vi "PFI-28000-Base_Get VISA.vi"(8 "error in (no error)":errorcluster, 11 "PFI-28000-Base in":refnum<class "PFI-28000-Base.lvclass">) -> (0 "error out":errorcluster, 2 "VISA":refnum<visa-resource-name>, 3 "PFI-28000-Base out":refnum<class "PFI-28000-Base.lvclass">)   [LabVIEW 2017, in "PFI-28000-Base.lvclass"]
uses:
  PFI-28000-Base.lvclass
  PFI-28000-Base.lvclass/PFI-28000-Base.ctl
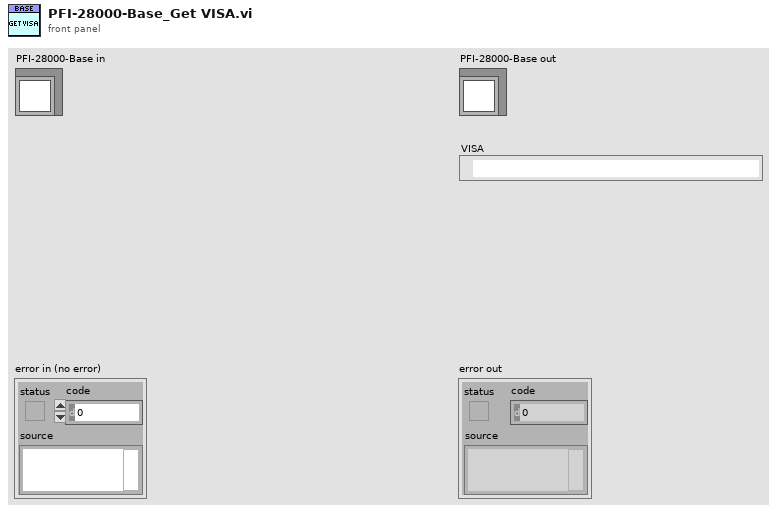
[diagram p1: front panel]
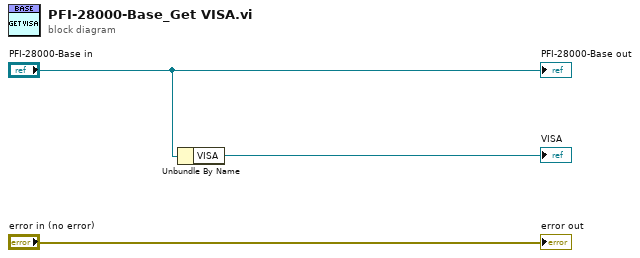
[diagram p0: block diagram]
diagram:
  n1 = Unbundle By Name("PFI-28000-Base in") -> ("VISA"=→"VISA":refnum<visa-resource-name>)
  "error out" <- "error in (no error)"
  "PFI-28000-Base out" <- "PFI-28000-Base in"
